vi "Mutate.TestStandTypePaletteFile.vi"(8 "error in (no error)":errorcluster, 11 "Version Build Information":T1={"VeriStand Version"="2013 SP1", "TestStand Version"="2013", "New VS Assembly Version"="2013.0.0.0", "New TS Assembly Version"="5.1.0.226", "VeriStand Steps Version String"="14.0.5.0", "Project Paths"={"MiscHelperVIs Project Path"="", "RTSequenceVIs Project Path"="", "Set Channels Project Path"="", "TS VS Logger Project Path"="", "VeriStand.exe Install Path"="", "NI_VeristandTypes.ini File Path"="", "Workspace Path"="", "VeristandSteps.csproj File Path"="", "Silent Veristand Project Path"=""}, "New TS Interop Assembly Version"="1.2.3.4", "New TS Utility Assembly Version"="5.6.7.8", "New VS Assembly Version (GAC)"="4.0.2016.0.9.9", "dotNET .config File Paths"={"MiscHelperVIs Project .config File Path"=path "C:/Users/Public/Documents/Git-Source/VeriStand-Custom-Steps-For-TestStand/Source/LabVIEW Code/Misc/MiscHelperVIs.lvproj.config", "RT Sequence VIs Project .config File Path"=path "C:/Users/Public/Documents/Git-Source/VeriStand-Custom-Steps-For-TestStand/Source/LabVIEW Code/RT Sequence/RTSequenceVIs.lvproj.config", "Set Channels Project .config File Path"=path "C:/Users/Public/Documents/Git-Source/VeriStand-Custom-Steps-For-TestStand/Source/LabVIEW Code/Set Channels/Set Channels.lvproj.config", "TS VS Logger Project .config File Path"=path "C:/Users/Public/Documents/Git-Source/VeriStand-Custom-Steps-For-TestStand/Source/LabVIEW Code/TS VS Logger/TS VS Logger.lvproj.config", "Silent Veristand Project .config File Path"=path "C:/Users/Public/Documents/Git-Source/VeriStand-Custom-Steps-For-TestStand/Source/LabVIEW Code/VeriStand Silent Start/SilentVS.lvproj.config"}}) -> (0 "error out":errorcluster, 3 "Version Build Information out":T1={"VeriStand Version"="2013 SP1", "TestStand Version"="2013", "New VS Assembly Version"="2013.0.0.0", "New TS Assembly Version"="5.1.0.226", "VeriStand Steps Version String"="14.0.5.0", "Project Paths"={"MiscHelperVIs Project Path"="", "RTSequenceVIs Project Path"="", "Set Channels Project Path"="", "TS VS Logger Project Path"="", "VeriStand.exe Install Path"="", "NI_VeristandTypes.ini File Path"="", "Workspace Path"="", "VeristandSteps.csproj File Path"="", "Silent Veristand Project Path"=""}, "New TS Interop Assembly Version"="1.2.3.4", "New TS Utility Assembly Version"="5.6.7.8", "New VS Assembly Version (GAC)"="4.0.2016.0.9.9", "dotNET .config File Paths"={"MiscHelperVIs Project .config File Path"=path "C:/Users/Public/Documents/Git-Source/VeriStand-Custom-Steps-For-TestStand/Source/LabVIEW Code/Misc/MiscHelperVIs.lvproj.config", "RT Sequence VIs Project .config File Path"=path "C:/Users/Public/Documents/Git-Source/VeriStand-Custom-Steps-For-TestStand/Source/LabVIEW Code/RT Sequence/RTSequenceVIs.lvproj.config", "Set Channels Project .config File Path"=path "C:/Users/Public/Documents/Git-Source/VeriStand-Custom-Steps-For-TestStand/Source/LabVIEW Code/Set Channels/Set Channels.lvproj.config", "TS VS Logger Project .config File Path"=path "C:/Users/Public/Documents/Git-Source/VeriStand-Custom-Steps-For-TestStand/Source/LabVIEW Code/TS VS Logger/TS VS Logger.lvproj.config", "Silent Veristand Project .config File Path"=path "C:/Users/Public/Documents/Git-Source/VeriStand-Custom-Steps-For-TestStand/Source/LabVIEW Code/VeriStand Silent Start/SilentVS.lvproj.config"}})   [LabVIEW 2014, in "VeriStand Steps Version Mutation.lvlib"]
uses:
  VeriStand Steps Version Mutation.lvlib
  Types/Version Build Information.ctl
  Types/Project Paths Cluster.ctl
  Types/dotNET Config File Paths Cluster.ctl
  <vilib>/xml/Load XML File.vi
  <vilib>/xml/Close Reference(Node).vi
  <vilib>/xml/Close Reference(NNMap).vi
  <resource>/objmgr/DOMUserDefRef.rc
  <vilib>/xml/NI_XML.lvlib
  <vilib>/ni/Simple XML/Simple XML.lvlib
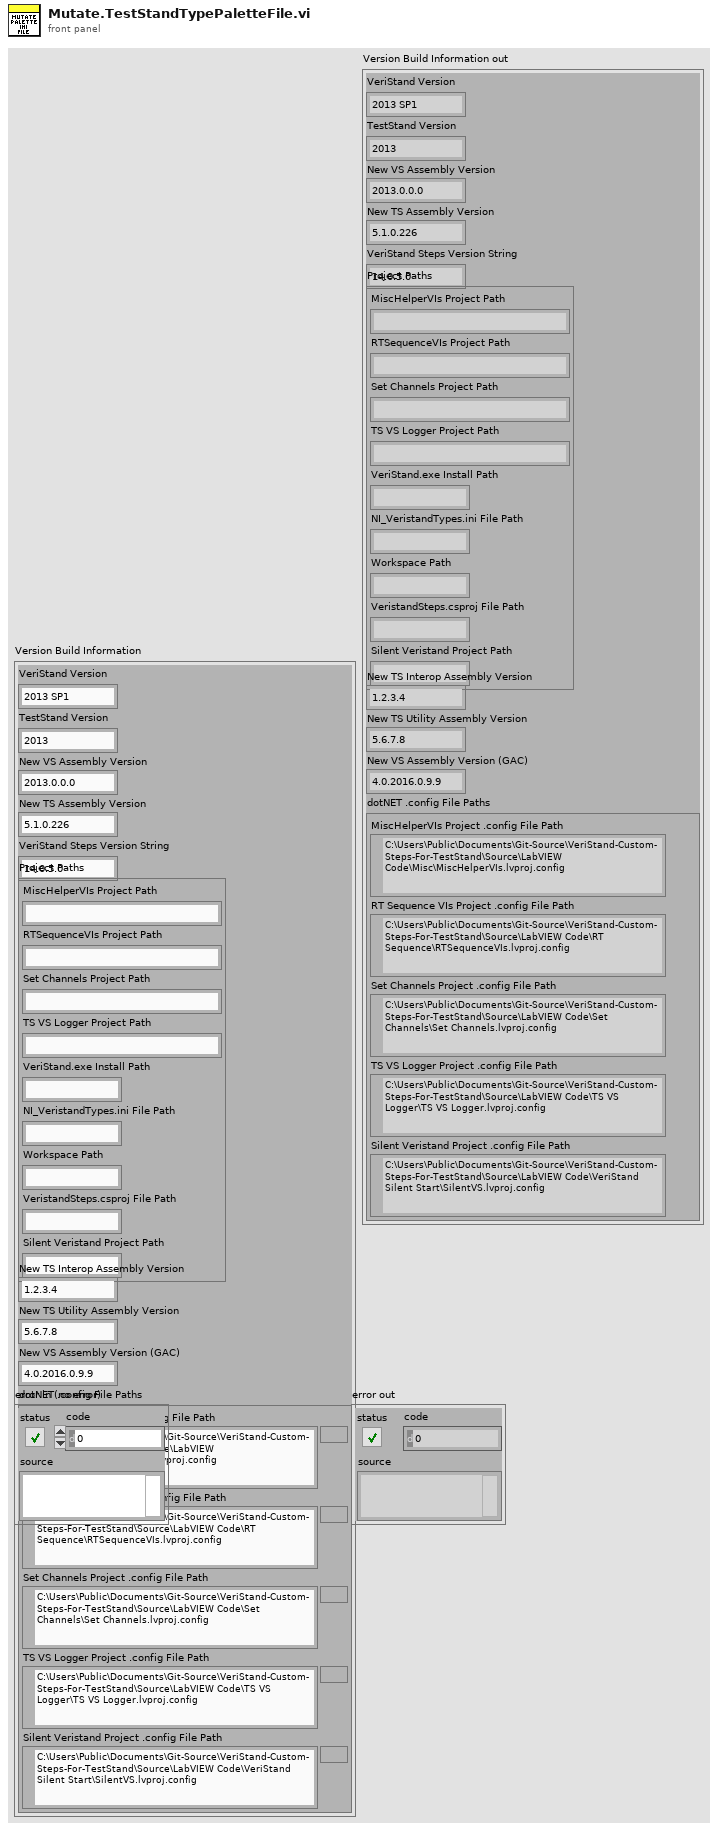
[diagram p1: front panel]
types:
  T1 = typedef "VeriStand Steps Version Mutation.lvlib/Version Build Information.ctl" = cluster{"VeriStand Version":string, "TestStand Version":string, "New VS Assembly Version":string, "New TS Assembly Version":string, "VeriStand Steps Version String":string, "Project Paths":T2, "New TS Interop Assembly Version":string, "New TS Utility Assembly Version":string, "New VS Assembly Version (GAC)":string, "dotNET .config File Paths":T3}
  T2 = typedef "VeriStand Steps Version Mutation.lvlib/Project Paths Cluster.ctl" = cluster{"MiscHelperVIs Project Path":string, "RTSequenceVIs Project Path":string, "Set Channels Project Path":string, "TS VS Logger Project Path":string, "VeriStand.exe Install Path":string, "NI_VeristandTypes.ini File Path":string, "Workspace Path":string, "VeristandSteps.csproj File Path":string, "Silent Veristand Project Path":string}
  T3 = typedef "VeriStand Steps Version Mutation.lvlib/dotNET Config File Paths Cluster.ctl" = cluster{"MiscHelperVIs Project .config File Path":path, "RT Sequence VIs Project .config File Path":path, "Set Channels Project .config File Path":path, "TS VS Logger Project .config File Path":path, "Silent Veristand Project .config File Path":path}
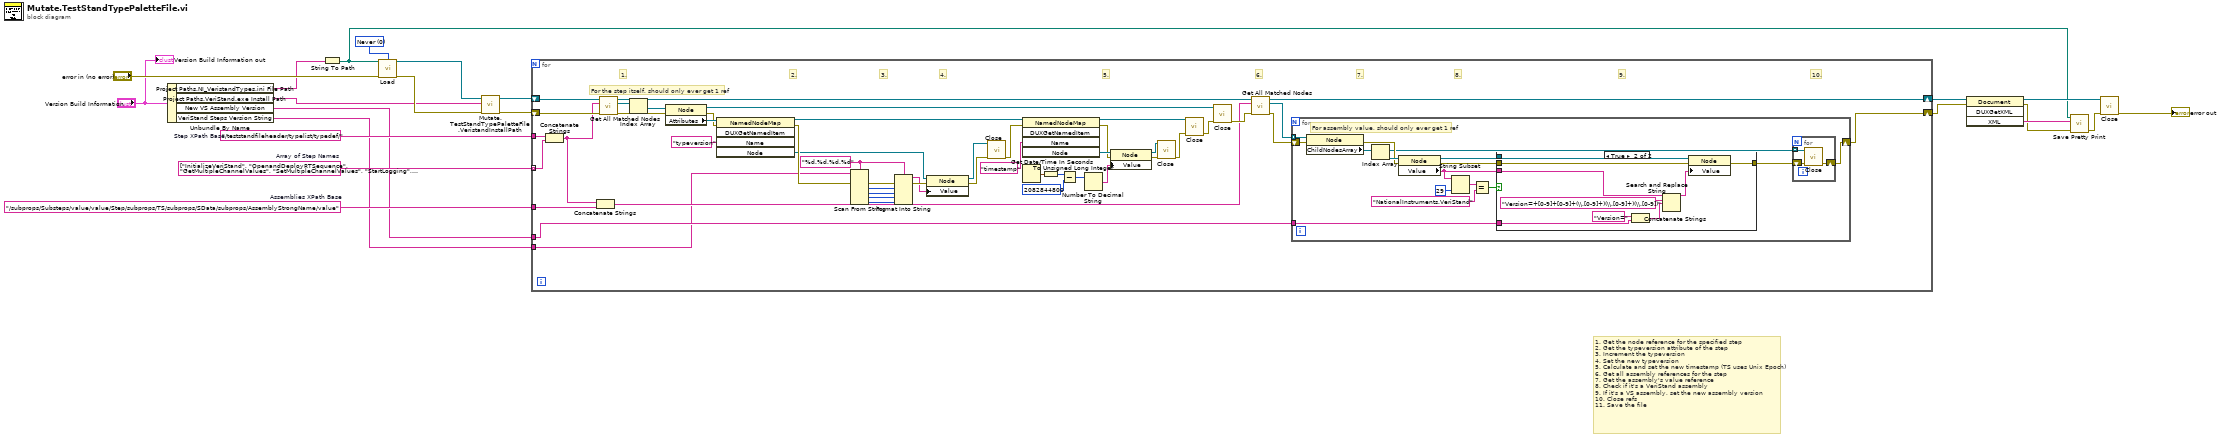
[diagram p0: block diagram]
diagram:
  w9 = "/subprops/Substeps/value/value/Step/subprops/TS/subprops/SData/subprops/AssemblyStrongName/value"  # Assemblies XPath Base
  w15 = string[] ["InitializeVeriStand", "OpenandDeployRTSequence", "GetMultipleChannelValues", "SetMultipleChannelValues", "StartLogging", "StopLogging", "StopVeriStand", "RunProject", "ConnectProject", "DisconnectProject", "UndeployProject", "RunStimulusProfileAsynch", "DeployProject", "OpenReferences", "GetAlarmState", "SetChannelValue", "GetAlarmList", "RunStimulusProfileBlocking", "SetAlarmState", "SetModelParameterValue", "CloseProject", "UpdateModelParametersFromFile", "GetChannelValue", "LimitTestChannelValue", "GetChannelFaultValue", "GetModelParameterValue", "ClearFault", "ClearAllFaults", "PauseRTSequence", "StopRTSequence", "GetSequenceState", "GetAllSequenceNames", "StartRTSequence", "AbortRTSequence", "GetSequenceReturnValue", "StartStimulusProfileSession", "RunRTSequenceAction", "CloseWorkspace", "OpenWorkspace", "SilentConnect", "SilentDisconnect", "OpenProject", "RunRTSequencePassFail", "RunRTSequenceNumericLimit", "SetChannelFaultValue", "StopVeristandGateway", "StartVeristand"]  # Array of Step Names
  w21 = "/teststandfileheader/typelist/typedef/"  # Step XPath Base
  w22 = 0 items=["Never", "Always", "Auto"] ("validate on load (Auto)")
  # "1. Get the node reference for the specified step\n2. Get the typeversion attribute of the step\n3. Increment the typeversion\n4. Set the new typeversion\n5. Calculate and set the new timestamp (TS uses Unix Epoch)\n6. Get all assembly references for the step\n7. Get the assembly's value reference\n8. Check if it's a VeriStand assembly\n9. If it's a VS assembly, set the new assembly version\n10. Close refs\n11. Save the file"
  n1 = Unbundle By Name("Version Build Information") -> ("Project Paths.NI_VeristandTypes.ini File Path"=w2:string, "Project Paths.VeriStand.exe Install Path"=w1:string, "New VS Assembly Version"=w3:string, "VeriStand Steps Version String"=w4:string)
  n2 = String To Path(string=w2) -> (path=w5:path)
  n3 = call-poly <vilib>:"Load.vi"("path to XML document"=w5, "validate on load (Auto)"=w22, "error in (no error)"="error in (no error)") -> ("DOM document out"=w13:refnum<k20>, "error out"=w14:errorcluster)  [unwired: 10 in, 1 out]
  n4 = call "Mutate.TestStandTypePaletteFile.VeristandInstallPath.vi"("error in (no error)"=w14, "New VS InstallPath"=w1, "DOM document in"=w13) -> ("error out"=w12:errorcluster, "DOM document out"=w11:refnum<k20>)  [unwired: 7 in]
  n5 = for {
    tunnel: w15 -> [w68] mode=indexing
    shift-right: [w66] -> w20
    shift-left: w11 -> [w71]
    tunnel: w21 -> [w69]
    shift-right: [w59] -> w10
    shift-left: w12 -> [w70]
    tunnel: w9 -> [w64]
    tunnel: w3 -> [w27]
    tunnel: w4 -> [w24]
    w48 = "%d.%d.%d.%d" ("format string")
    # "10."
    # "9."
    # "8."
    # "7."
    # "6."
    # "5."
    # "4."
    # "3."
    # "2."
    # "1."
    # "For the step itself, should only ever get 1 ref"
    n6 = Concatenate Strings(w69, w68) -> (w63:string)
    n7 = Concatenate Strings(w63, w64) -> (w62:string)
    n8 = call <vilib>:"Get All Matched Nodes.vi"("error in (no error)"=w70, "XPath expression"=w63, "node in"=w71) -> ("error out"=w54:errorcluster, "node result array"=w58:refnum<k20>[], "node out"=w67:refnum<k20>)  [unwired: 6 in]
    n9 = Index Array(array=w58) -> (element=w57:refnum<k20>)  [unwired: 1 in]
    n10 = property class="Node"(reference=w57, error in=w54) -> (reference out=w32:refnum<k20>, error out=w55:errorcluster, "Attributes"=w56:refnum<k20>)
    n11 = invoke class="NamedNodeMap" method="DUXGetNamedItem"(reference=w56, error in=w55, "Name"="typeversion") -> (reference out=w47:refnum<k20>, error out=w25:errorcluster, "Node"=w23:refnum<k20>)  [unwired: 2 in, 2 out]
    n12 = Scan From String(format string=w48, input string=w24, error in=w25) -> (error out=w52:errorcluster, output 1=w51:i32, output 2=w50:i32, output 3=w49:i32, output 4=w26:i32)  [unwired: 5 in, 2 out]
    n13 = Format Into String(format string=w48, error in=w52, w51, w50, w49, w26) -> (resulting string=w45:string, error out=w46:errorcluster)  [unwired: 1 in]
    n14 = property class="Node"(reference=w23, error in=w46, "Value"=w45) -> (reference out=w43:refnum<k20>, error out=w44:errorcluster)
    n15 = call-poly <vilib>:"Close.vi"("error in (no error)"=w44, "node"=w43) -> ("error out"=w42:errorcluster)  [unwired: 7 in]
    n16 = invoke class="NamedNodeMap" method="DUXGetNamedItem"(reference=w47, error in=w42, "Name"="timestamp") -> (reference out=w35:refnum<k20>, error out=w39:errorcluster, "Node"=w40:refnum<k20>)  [unwired: 2 in, 2 out]
    n17 = Get Date/Time In Seconds() -> (seconds since 1Jan1904=w31:timestamp)
    n18 = To Unsigned Long Integer(number=w31) -> (unsigned 32bit integer=w30:u32)
    n19 = Subtract(x=w30, y=u32 2082844800) -> (x-y=w28:u32)
    n20 = Number To Decimal String(number=w28) -> (decimal integer string=w38:string)  [unwired: 1 in]
    n21 = property class="Node"(reference=w40, error in=w39, "Value"=w38) -> (reference out=w36:refnum<k20>, error out=w37:errorcluster)
    n22 = call-poly <vilib>:"Close.vi"("error in (no error)"=w37, "node"=w36) -> ("error out"=w34:errorcluster)  [unwired: 7 in]
    n23 = call-poly <vilib>:"Close.vi"("error in (no error)"=w34, "named node map"=w35) -> ("error out"=w33:errorcluster)  [unwired: 7 in]
    n24 = call-poly <vilib>:"Close.vi"("error in (no error)"=w33, "node"=w32) -> ("error out"=w65:errorcluster)  [unwired: 7 in]
    n25 = call <vilib>:"Get All Matched Nodes.vi"("error in (no error)"=w65, "XPath expression"=w62, "node in"=w67) -> ("error out"=w60:errorcluster, "node result array"=w61:refnum<k20>[], "node out"=w66:refnum<k20>)  [unwired: 6 in]
    n26 = for {
      tunnel: w61 -> [w86] mode=indexing
      shift-right: [w81] -> w59
      shift-left: w60 -> [w85]
      tunnel: w27 -> [w72]
      # "For assembly value, should only ever get 1 ref"
      n27 = property class="Node"(reference=w86, error in=w85) -> (error out=w83:errorcluster, "ChildNodesArray"=w82:refnum<k20>[])  [unwired: 1 out]
      n28 = Index Array(array=w82) -> (element=w84:refnum<k20>)  [unwired: 1 in]
      n29 = property class="Node"(reference=w84, error in=w83) -> (reference out=w78:refnum<k20>, error out=w79:errorcluster, "Value"=w77:string)
      n30 = String Subset(string=w77, length (rest)=29 ("length (rest)")) -> (substring=w75:string)  [unwired: 1 in]
      n31 = Equal?(x=w75, y="NationalInstruments.VeriStand" ("Node Value 2")) -> (x = y?=w73:bool)
      n32 = case shown="True" w73 {
        tunnel: w77 -> [_ w96]
        tunnel: [w87 w92] -> w80
        tunnel: w79 -> [w87 w90]
        tunnel: w78 -> [_ w89]
        tunnel: w72 -> [_ w88]
        frame False {
        }
        frame True {
          n33 = Concatenate Strings("Version=" ("replace string (\"\")"), w88) -> (w93:string)
          n34 = Search and Replace String(input string=w96, search string="Version=+[0-9]+[0-9]+(\\.[0-9]+)(\\.[0-9]+)(\\.[0-9])", replace string=w93) -> (result string=w91:string)  [unwired: 5 in, 3 out]
          n35 = property class="Node"(reference=w89, error in=w90, "Value"=w91) -> (error out=w92:errorcluster)  [unwired: 1 out]
        }
      }
      n36 = for {
        tunnel: w82 -> [w99] mode=indexing
        shift-right: [w97] -> w81
        shift-left: w80 -> [w98]
        n37 = call-poly <vilib>:"Close.vi"("error in (no error)"=w98, "node"=w99) -> ("error out"=w97:errorcluster)  [unwired: 7 in]
      }
    }
  }
  n38 = invoke class="Document" method="DUXGetXML"(reference=w20, error in=w10) -> (reference out=w17:refnum<k20>, error out=w18:errorcluster, "XML"=w19:string)  [unwired: 2 in, 1 out]
  n39 = call <vilib>:"Save Pretty Print.vi"("error in (no error)"=w18, "Pretty XML String"=w19, "XML file path"=w5) -> ("error out"=w16:errorcluster)  [unwired: 7 in, 1 out]
  n40 = call-poly <vilib>:"Close.vi"("error in (no error)"=w16, "node"=w17) -> ("error out"=→"error out":errorcluster)  [unwired: 7 in]
  "Version Build Information out" <- "Version Build Information"
